vi "StateMachine_Global.vi"() -> ()   [LabVIEW 2019]
panel:
  out "Hood Shooter Setpoint":dbl
  out "Hood Setpoint":dbl
  out "Shooter Setpoint":dbl
  out "Turret Free Mode":bool
  in  "Dragoon Mode":bool
  out "Encoder?":bool
  out "Turn LL ON":bool
  out "Turret Setpoint":dbl
  out "ClimberPull":bool
  out "ClimberOutput":dbl
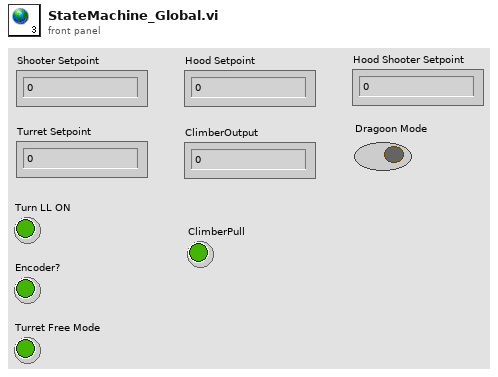
[diagram p1: front panel]
diagram:
